vi "Divider0.vi"() -> (8 "Divider0":refnum<class "Divider0.lvclass">)   [LabVIEW 2017, in "Divider0.lvclass"]
uses:
  Divider0.lvclass
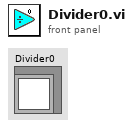
[diagram p1: front panel]
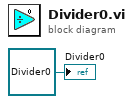
[diagram p0: block diagram]
diagram:
  "Divider0" <- refnum<class "Divider0.lvclass"> refnum ("Divider0.lvclass")
